vi "PSUN8731A-CTRLv3.vi"() -> ()   [LabVIEW 2017]
uses:
  Keysight N8731A conversion/Keysight N8900 Series.lvlib
  Controller subVIs/CurrentPSUSettings.vi
  <vilib>/Analysis/NI_AALPro.lvlib
  <vilib>/Analysis/6fits.llb/Curve Fitting Criteria.ctl
panel:
  in  "Quench Protection":bool
  out "Status message":string
  out "TimeData":dbl[](array[numeric])
  out "VoltData":dbl[](array[numeric])
  out "CurrData":dbl[](array[numeric])
  out "StartTime":dbl
  out "I(t)":cluster{dbl[], dbl[]}(graph)
  out "V(t)":cluster{dbl[], dbl[]}(graph)
  in  "Sweep Controller":enum32{"Sweep Mode", "Free Control Mode"}(tab)=enum."Free Control Mode"
  in  "Maximum Voltage [V]":dbl min=0.0 max=8.0 step=0.001
  in  "Maximum Current [A]":dbl min=0.0 max=400.0 step=0.1
  in  "Coil Voltage Limit [V]":dbl=0.005 min=0.0 step=0.001
  in  "Initial Voltage [V]":dbl min=0.0 max=8.0 step=0.001
  in  "Initial meas delay [ms]":u32=500 step=10
  in  "Tr meas time [s]":dbl=60.0 min=0.0
  out "Voltage offset [V]":dbl
  out "Tr [s]":dbl
  in  "Time between data points (ms)":i32=500 min=0
  out "Immediate Voltage (V)":dbl
  out "Immediate Current (A)":dbl
  in  "Voltage Set [V]":dbl min=0.0 max=8.0 step=0.001
  in  "Current Set [A]":dbl min=0.0 max=400.0 step=0.1
  in  "Voltmeter channel (6)":i32=6
  in  "End Program":bool
  in  "Stop Sweep":bool
  out "Voltmeter error message":errorcluster
  in  "Voltmeter Range (V)":dbl caption="0 for Auto range"
  in  "Voltmeter Address (16)":i16=16
  out "PSU error message":errorcluster
  in  "Start Sweep":bool
  in  "Sweepback":bool=TRUE
  in  "Power Output":bool
  in  "OC protection":bool
  in  "OV Value (10V)":dbl=10.0 min=0.5 max=10.0
  out "I(V) Graph":cluster{dbl[], dbl[]}(graph)
  in  "VISA resource name":refnum<visa-resource-name>="N8731APSU"
  in  "Filename":string caption="Leave empty to discard data.\nDon't touch during measurement"
  in  "PSU\nVoltage":bool=TRUE caption="Keithley\nVoltage"
  in  "OV protection":bool=TRUE
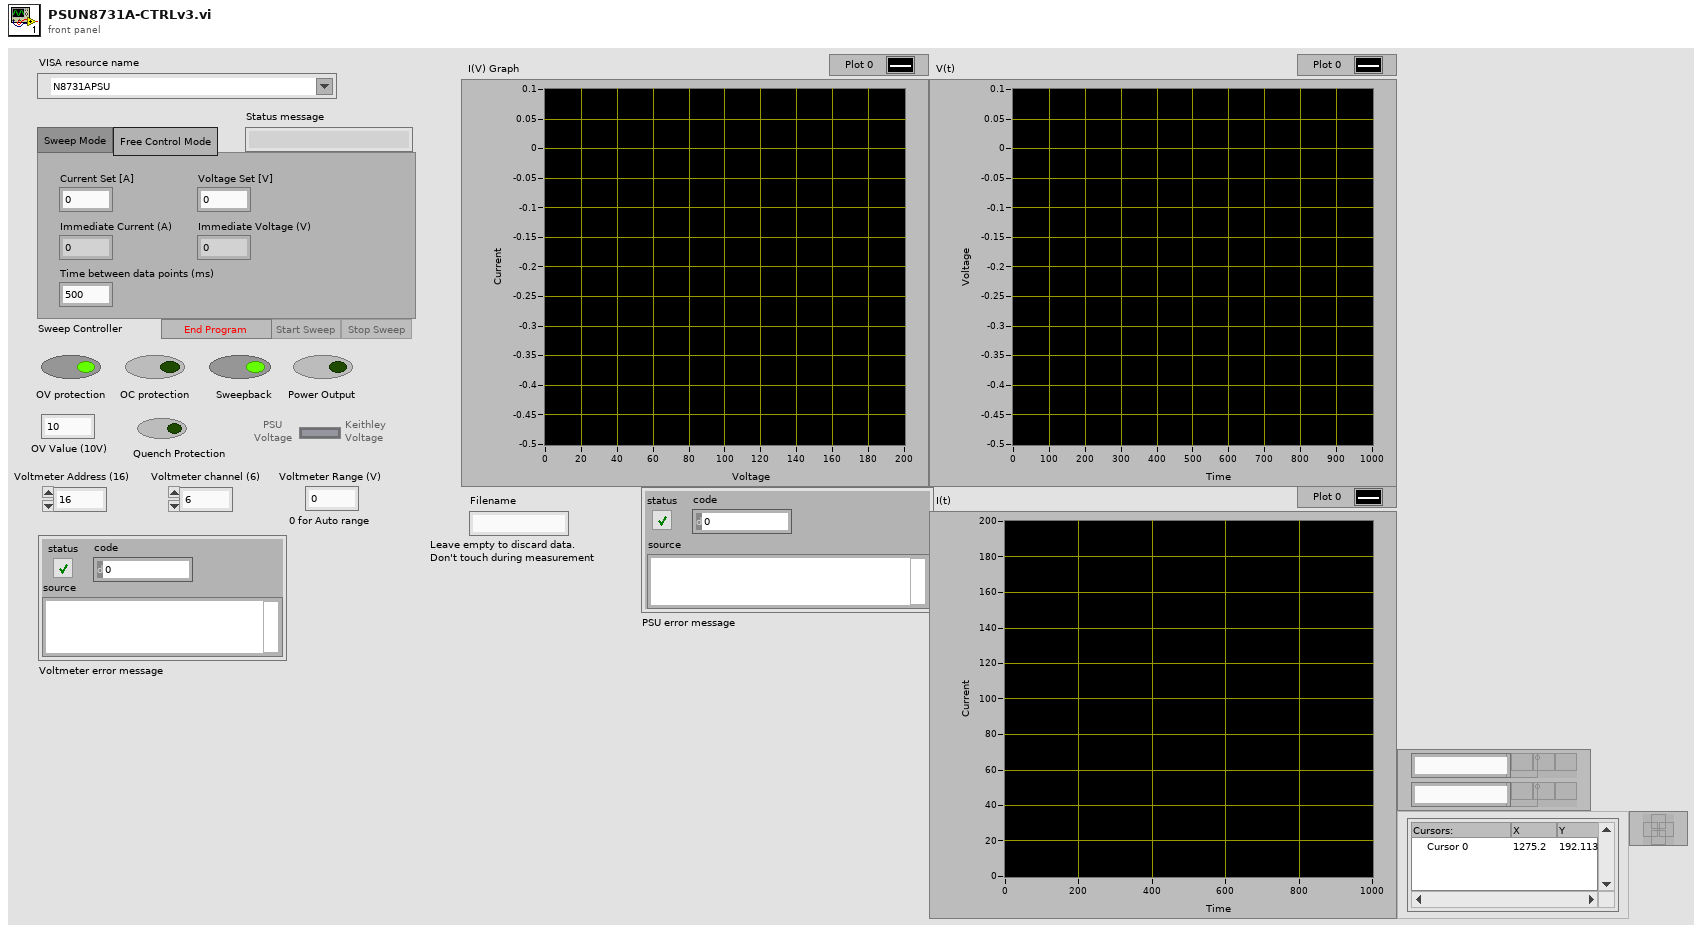
[diagram p1: front panel]
types:
  T1 = enum8{"Enabled", "Disabled", "Disabled and Grayed Out"}
  T2 = cluster{"Sweep Controller":enum32{"Sweep Mode", "Free Control Mode"}, "   PSU\nVoltage":bool}
  T3 = typedef "NI_AALPro.lvlib/Curve Fitting Criteria.ctl" = u16
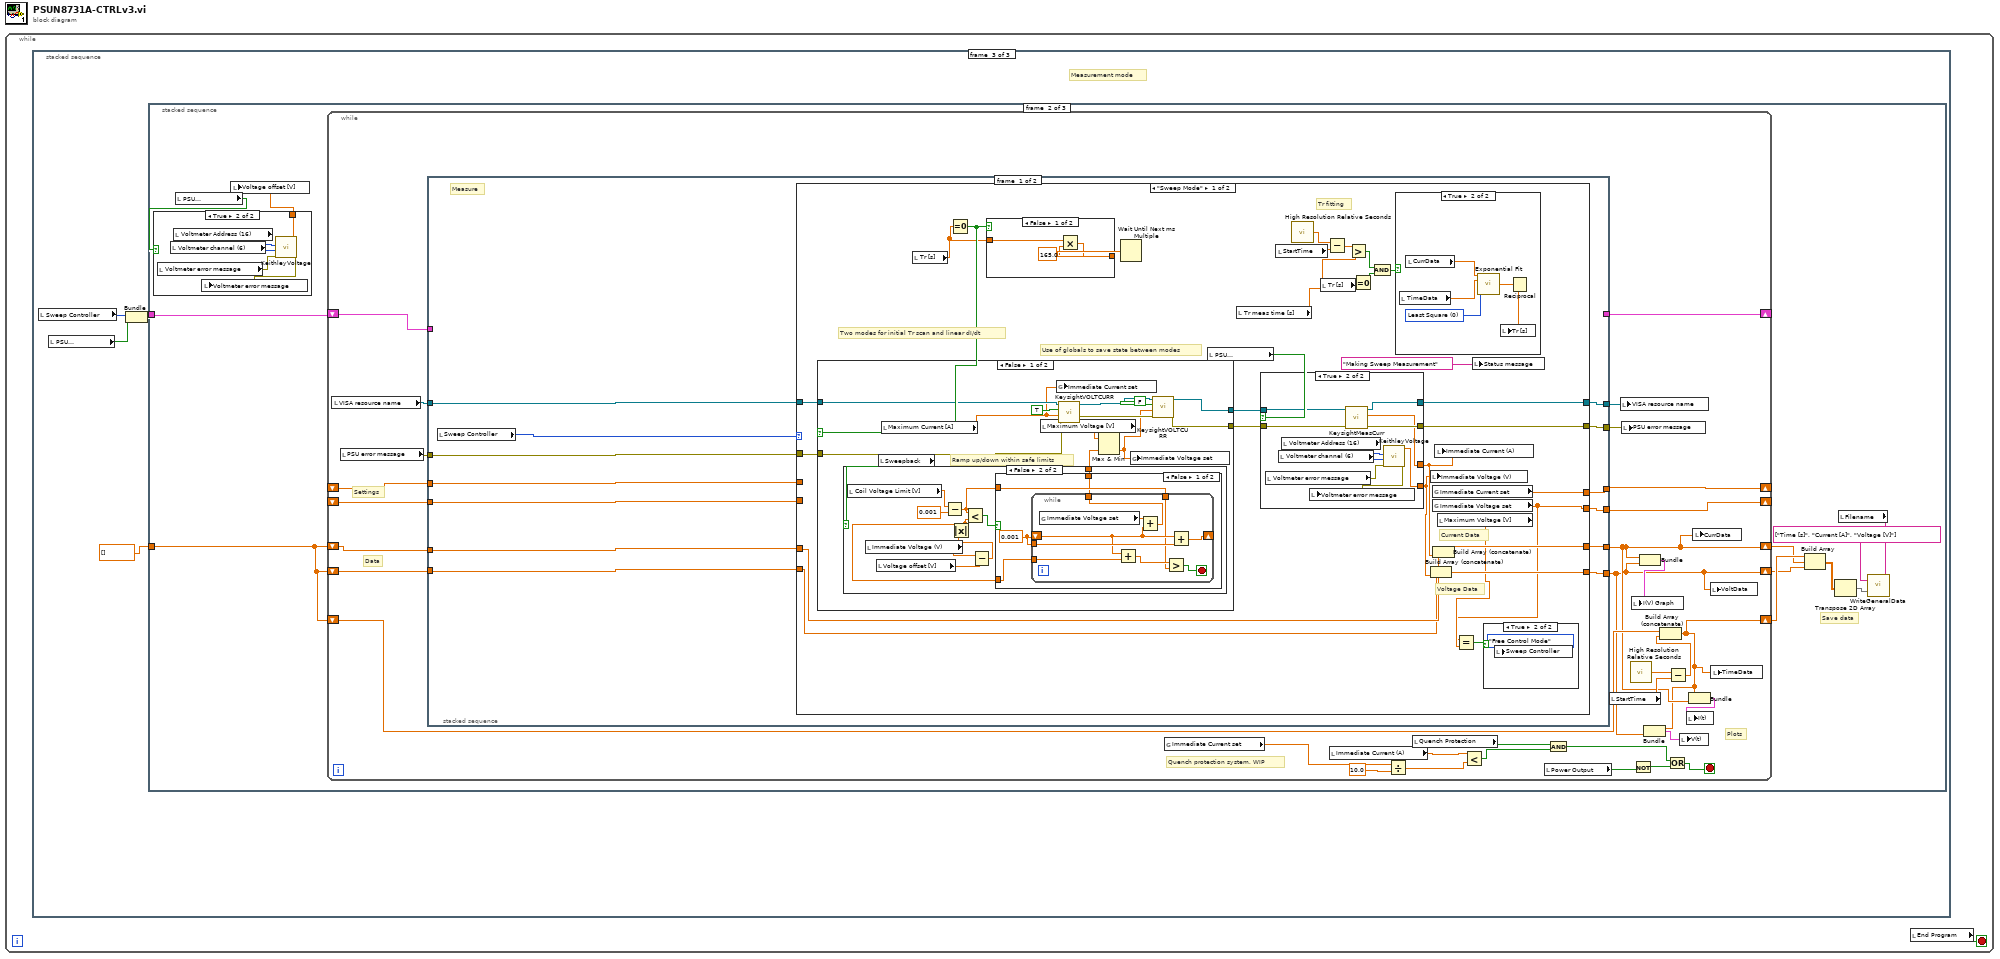
[diagram p0: block diagram]
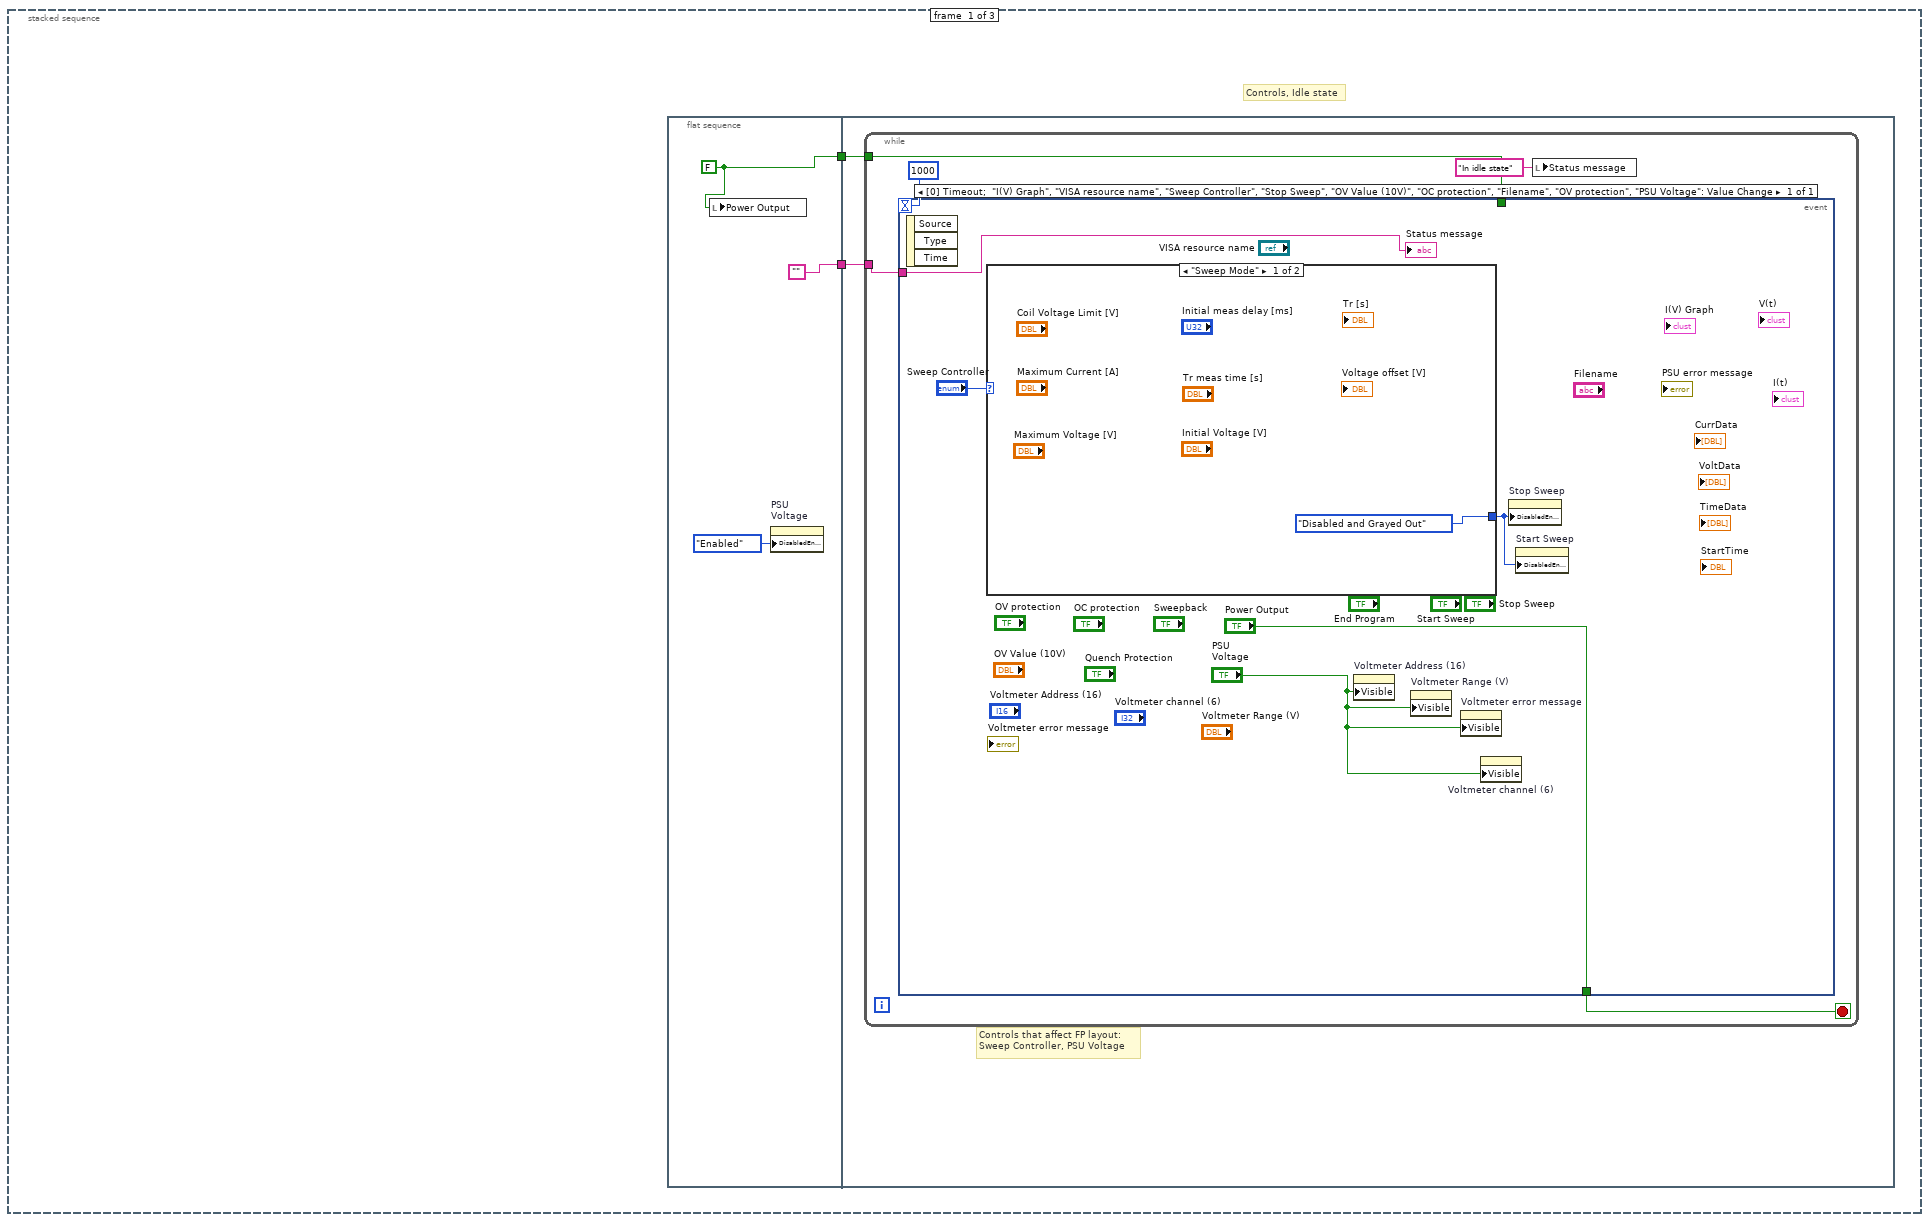
[diagram p2: hidden frame]
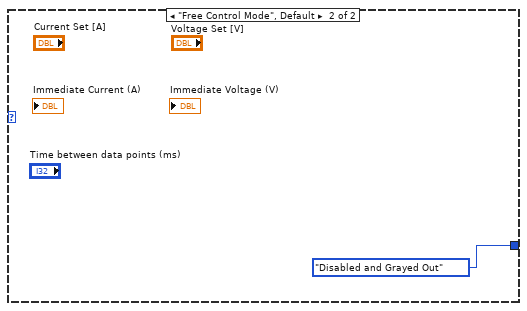
[diagram p3: hidden frame]
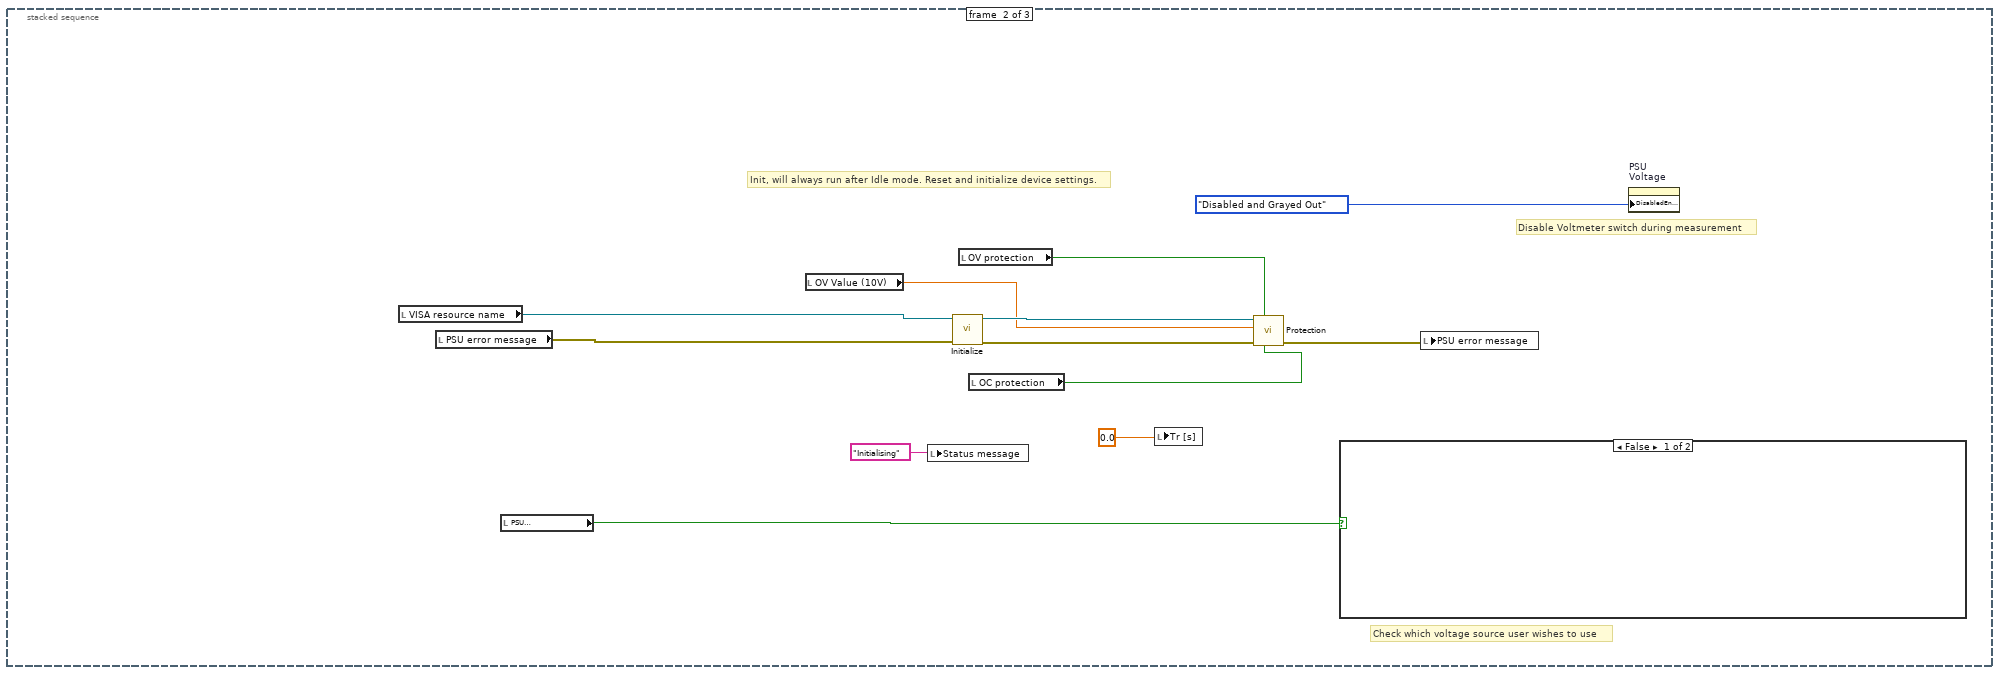
[diagram p4: hidden frame]
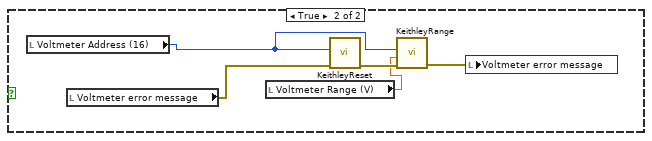
[diagram p5: hidden frame]
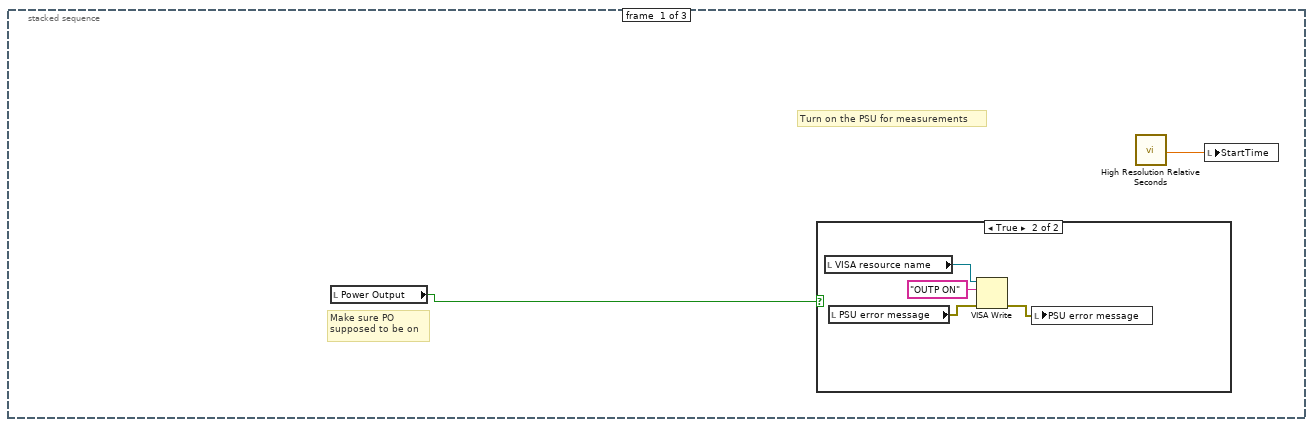
[diagram p6: hidden frame]
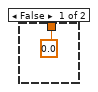
[diagram p8: hidden frame]
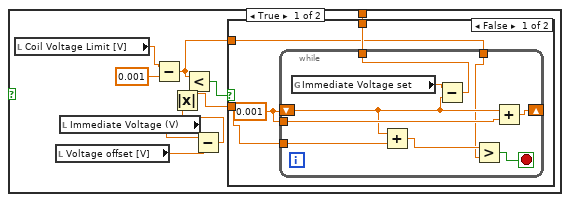
[diagram p10: hidden frame]
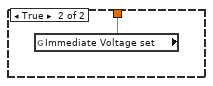
[diagram p11: hidden frame]
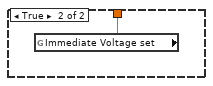
[diagram p12: hidden frame]
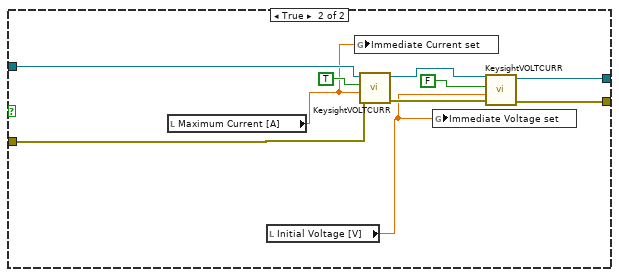
[diagram p13: hidden frame]
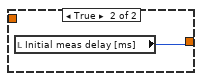
[diagram p15: hidden frame]
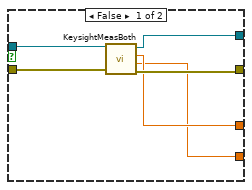
[diagram p16: hidden frame]
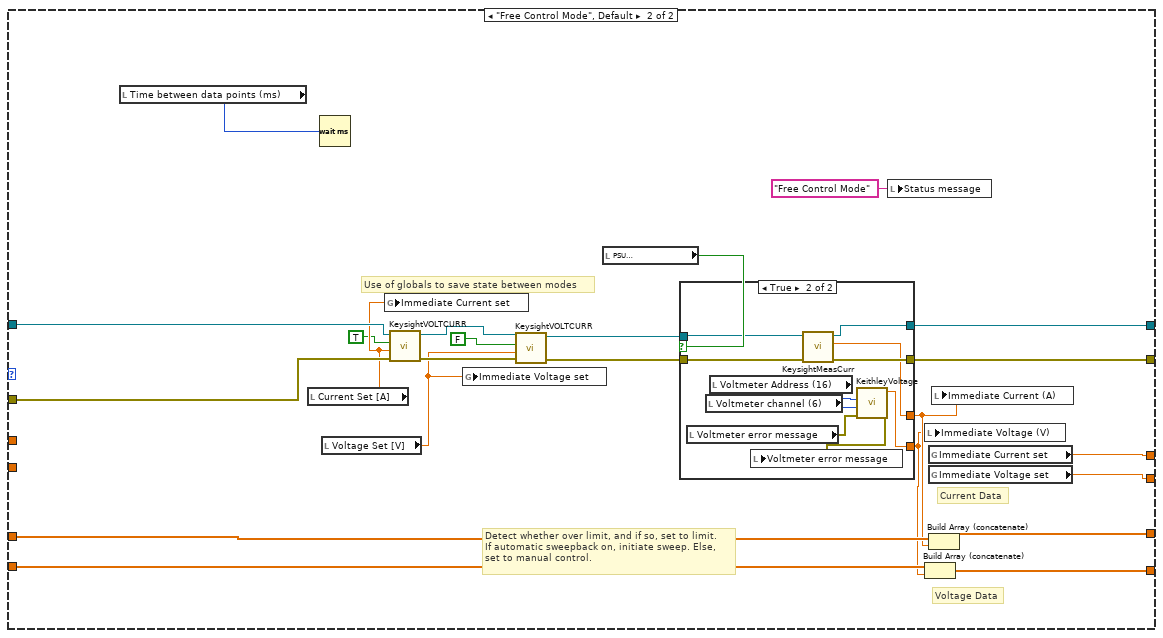
[diagram p17: hidden frame]
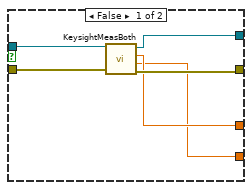
[diagram p18: hidden frame]
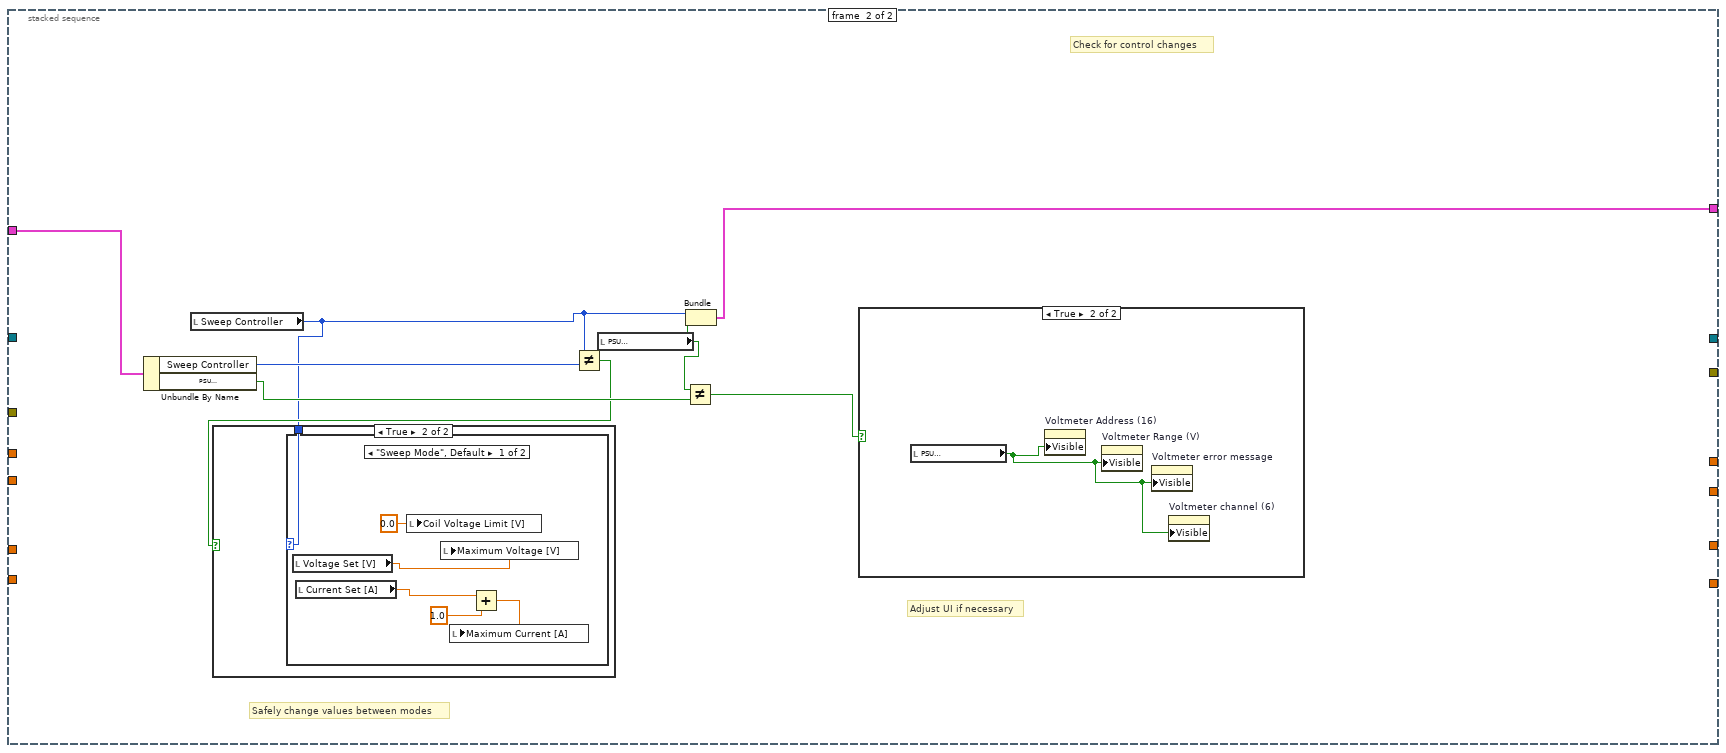
[diagram p19: hidden frame]
diagram:
  n1 = while {
    stop <- w1 stop-if-true
    n2 = stacked-sequence {
      frame #0 {
        # "Controls, Idle state"
        n3 = flat-sequence {
          tunnel: [w4] -> w3
          tunnel: ["" ("Status message")] -> w2
          tunnel: w3 -> [w8]
          tunnel: w2 -> [w7]
          frame #0 {
            w4 = FALSE ("Sweeping Back")
            n4 = local write "Power Output"(w4) -> ()
            n5 = property on="PSU\nVoltage" class="Bool (strict)"("DisabledEnum"=T1."Enabled" ("Disabled")) -> ()  [unwired: 2 in, 2 out]
          }
          frame #1 {
            # "Controls that affect FP layout:\nSweep Controller, PSU Voltage"
            n6 = while {
              tunnel: w8 -> [w11]
              tunnel: w7 -> [w10]
              stop <- w13 stop-if-true
              n7 = event shown="[0] Timeout;  \"I(V) Graph\", \"VISA resource name\", \"Sweep Controller\", \"Stop Sweep\", \"OV Value (10V)\", \"OC protection\", \"Filename\", \"OV protection\", \"PSU Voltage\": Value Change" {
                selector: _ -> [_]
                dyn-events: _ -> [_]
                timeout: 1000 -> [_]
                tunnel: ["Power Output"] -> w13
                tunnel: w11 -> [w16]
                tunnel: w10 -> [w14]
                event Timeout; "I(V) Graph", "VISA resource name", "Sweep Controller", "Stop Sweep", "OV Value (10V)", "OC protection", "Filename", "OV protection", "PSU\nVoltage": Value Change {
                  n8 = event-data() -> ()  [unwired: 1 in, 3 out]
                  n9 = case shown="\"Sweep Mode\"" "Sweep Controller" {
                    tunnel: [T1."Disabled and Grayed Out" ("Disabled") T1."Disabled and Grayed Out" ("Disabled")] -> w17
                    frame "Sweep Mode" {
                    }
                    frame "Free Control Mode", Default {
                    }
                  }
                  n10 = property on="Voltmeter Address (16)" class="DigNum (strict)"("Visible"="PSU\nVoltage") -> ()  [unwired: 2 in, 2 out]
                  n11 = property on="Voltmeter Range (V)" class="DigNum (strict)"("Visible"="PSU\nVoltage") -> ()  [unwired: 2 in, 2 out]
                  n12 = property on="Voltmeter error message" class="Clust (strict)"("Visible"="PSU\nVoltage") -> ()  [unwired: 2 in, 2 out]
                  n13 = property on="Voltmeter channel (6)" class="DigNum (strict)"("Visible"="PSU\nVoltage") -> ()  [unwired: 2 in, 2 out]
                  n14 = property on="Stop Sweep" class="Bool"("DisabledEnum"=w17) -> ()  [unwired: 2 in, 2 out]
                  n15 = property on="Start Sweep" class="Bool"("DisabledEnum"=w17) -> ()  [unwired: 2 in, 2 out]
                  "Status message" <- w14
                }
              }
              n16 = local write "Status message"("In idle state" ("Status message")) -> ()
            }
          }
        }
      }
      frame #1 {
        # "Check which voltage source user wishes to use"
        # "Disable Voltmeter switch during measurement"
        # "Init, will always run after Idle mode. Reset and initialize device settings."
        n17 = local read "VISA resource name"() -> (w31:refnum<visa-resource-name>)
        n18 = local read "PSU error message"() -> (w26:errorcluster)
        n19 = local read "PSU\nVoltage"() -> (w25:bool)
        n20 = local read "OV Value (10V)"() -> (w30:dbl)
        n21 = local write "Status message"("Initialising" ("Status message")) -> ()
        n22 = call "Initialize.vi"("error in (no error)"=w26, "VISA resource name"=w31) -> ("error out"=w32:errorcluster, "VISA resource name out"=w33:refnum<visa-resource-name>)  [unwired: 8 in]
        n23 = local read "OV protection"() -> (w28:bool)
        n24 = local read "OC protection"() -> (w29:bool)
        n25 = local write "Tr [s]"(0.0 ("Tr")) -> ()
        n26 = call "Protection.vi"("OC protection"=w29, "OV protection"=w28, "error in (no error)"=w32, "OV Value (10V)"=w30, "VISA resource name"=w33) -> ("error out"=w27:errorcluster)  [unwired: 5 in, 1 out]
        n27 = case shown="False" w25 {
          frame False {
          }
          frame True {
            n28 = local read "Voltmeter Address (16)"() -> (w34:i16)
            n29 = local read "Voltmeter error message"() -> (w36:errorcluster)
            n30 = local read "Voltmeter Range (V)"() -> (w35:dbl)
            n31 = call "KeithleyReset.vi"("error in"=w36, "address (16)"=w34) -> ("error out"=w37:errorcluster)  [unwired: 9 in]
            n32 = call "KeithleyRange.vi"("error in"=w37, "Range (V)/Auto(0)"=w35, "address (16)"=w34) -> ("error out"=w38:errorcluster)  [unwired: 8 in]
            n33 = local write "Voltmeter error message"(w38) -> ()
          }
        }
        n34 = local write "PSU error message"(w27) -> ()
        n35 = property on="PSU\nVoltage" class="Bool (strict)"("DisabledEnum"=T1."Disabled and Grayed Out" ("Disabled")) -> ()  [unwired: 2 in, 2 out]
      }
      frame #2 {
        # "Measurement mode"
        n36 = local read "Sweep Controller"() -> (w42:enum32{"Sweep Mode", "Free Control Mode"})
        n37 = local read "PSU\nVoltage"() -> (w41:bool)
        n38 = Bundle("Sweep Controller"=w42, "PSU\nVoltage"=w41) -> (w40:T2)  [unwired: 1 in]
        n39 = stacked-sequence {
          tunnel: w40 -> [_ w59 _]
          tunnel: dbl[] [] -> [_ w58 _]
          frame #0 {
            # "Make sure PO\nsupposed to be on"
            # "Turn on the PSU for measurements"
            n40 = local read "Power Output"() -> (w44:bool)
            n41 = case shown="True" w44 {
              frame False {
              }
              frame True {
                n42 = local read "VISA resource name"() -> (w47:refnum<visa-resource-name>)
                n43 = local read "PSU error message"() -> (w46:errorcluster)
                n44 = VISA Write(VISA resource name=w47, write buffer="OUTP ON", error in (no error)=w46) -> (error out=w45:errorcluster)  [unwired: 2 out]
                n45 = local write "PSU error message"(w45) -> ()
              }
            }
            n46 = call <vilib>:"High Resolution Relative Seconds.vi"() -> ("relative seconds"=w43:dbl)
            n47 = local write "StartTime"(w43) -> ()
          }
          frame #1 {
            # "Save data"
            n48 = local read "PSU\nVoltage"() -> (w57:bool)
            n49 = case shown="True" w57 {
              tunnel: [0.0 ("Voltage") w61] -> w56
              frame False {
              }
              frame True {
                n50 = local read "Voltmeter error message"() -> (w63:errorcluster)
                n51 = local read "Voltmeter channel (6)"() -> (w65:i32)
                n52 = local read "Voltmeter Address (16)"() -> (w64:i16)
                n53 = call "KeithleyVoltage.vi"("error in"=w63, "channel (6)"=w65, "address (16)"=w64) -> ("error out"=w62:errorcluster, "Voltage"=w61:dbl)  [unwired: 7 in]
                n54 = local write "Voltmeter error message"(w62) -> ()
              }
            }
            n55 = local write "Voltage offset [V]"(w56) -> ()
            n56 = while {
              shift-right: [w67] -> _
              shift-left: w59 -> [w97]
              shift-right: [w88] -> _
              shift-left: _ -> [w86]
              shift-right: [w89] -> _
              shift-left: _ -> [w94]
              shift-right: [w70] -> w52
              shift-left: w58 -> [w91]
              shift-right: [w69] -> w51
              shift-left: w58 -> [w90]
              shift-right: [w68] -> w53
              shift-left: w58 -> [w84]
              stop <- w71 stop-if-true
              # "Plots"
              # "Quench protection system, WIP"
              # "Data"
              # "Settings"
              n57 = local read "VISA resource name"() -> (w96:refnum<visa-resource-name>)
              n58 = local read "PSU error message"() -> (w95:errorcluster)
              n59 = stacked-sequence {
                tunnel: w97 -> [_ w280]
                tunnel: w96 -> [w109 _]
                tunnel: w95 -> [w108 _]
                tunnel: w94 -> [w107 _]
                tunnel: [w106 _] -> w93
                tunnel: [w105 _] -> w92
                tunnel: w91 -> [w104 _]
                tunnel: [w103 _] -> w70
                tunnel: w90 -> [w102 _]
                tunnel: [w101 _] -> w69
                tunnel: [w100 _] -> w89
                tunnel: [w99 _] -> w88
                tunnel: w86 -> [w98 _]
                tunnel: [_ w276] -> w67
                frame #0 {
                  # "Measure"
                  n60 = local read "Sweep Controller"() -> (w110:enum32{"Sweep Mode", "Free Control Mode"})
                  n61 = case shown="\"Sweep Mode\"" w110 {
                    tunnel: w109 -> [w139 w257]
                    tunnel: w108 -> [w138 w256]
                    tunnel: w107 -> [_ _]
                    tunnel: [w137 w255] -> w106
                    tunnel: [w136 w254] -> w105
                    tunnel: w104 -> [w135 w253]
                    tunnel: [w134 w252] -> w103
                    tunnel: w102 -> [w117 w251]
                    tunnel: [w133 w250] -> w101
                    tunnel: [w127 w238] -> w100
                    tunnel: [w111 w237] -> w99
                    tunnel: w98 -> [_ _]
                    frame "Sweep Mode" {
                      # "Tr fitting"
                      # "Two modes for initial Tr scan and linear dI/dt"
                      # "Use of globals to save state between modes"
                      # "Voltage Data"
                      # "Current Data"
                      n62 = local read "Tr [s]"() -> (w116:dbl)
                      n63 = Equal To 0?(x=w116) -> (x = 0?=w118:bool)
                      n64 = case shown="False" w118 {
                        tunnel: w139 -> [w153 w209]
                        tunnel: w138 -> [w152 w208]
                        tunnel: [w147 w203] -> w131
                        tunnel: [w146 w202] -> w130
                        frame False {
                          # "Ramp up/down within safe limits"
                          n65 = local read "Sweepback"() -> (w144:bool)
                          n66 = case shown="False" w144 {
                            tunnel: [w162 w185] -> w142
                            frame True {
                              n67 = local read "Coil Voltage Limit [V]"() -> (w157:dbl)
                              n68 = local read "Voltage offset [V]"() -> (w160:dbl)
                              n69 = local read "Immediate Voltage (V)"() -> (w161:dbl)
                              n70 = Subtract(x=w157, y=0.001) -> (x-y=w155:dbl)
                              n71 = Subtract(x=w161, y=w160) -> (x-y=w156:dbl)
                              n72 = Absolute Value(x=w156) -> (abs(x)=w154:dbl)
                              n73 = Less?(x=w155, y=w154) -> (x < y?=w159:bool)
                              n74 = case shown="False" w159 {
                                tunnel: [w165 w176] -> w162
                                tunnel: w155 -> [w164 _]
                                tunnel: w154 -> [w163 _]
                                frame False {
                                w166 = 0.001 ("y")
                                n75 = while {
                                shift-right: [w174] -> _
                                shift-left: w166 -> [w169]
                                tunnel: w166 -> [w173]
                                tunnel: [w172] -> w165
                                tunnel: w164 -> [w167]
                                tunnel: w163 -> [w170]
                                stop <- w175 stop-if-true
                                n76 = global read "CurrentPSUSettings.vi" "Immediate Voltage set"() -> (w171:dbl)
                                n77 = Add(x=w169, y=w170) -> (x+y=w168:dbl)
                                n78 = Subtract(x=w171, y=w169) -> (x-y=w172:dbl)
                                n79 = Greater?(x=w168, y=w167) -> (0:w175:bool)
                                n80 = Add(x=w169, y=w173) -> (x+y=w174:dbl)
                                }
                                }
                                frame True {
                                n81 = global read "CurrentPSUSettings.vi" "Immediate Voltage set"() -> (w176:dbl)
                                }
                              }
                            }
                            frame False {
                              n82 = local read "Coil Voltage Limit [V]"() -> (w180:dbl)
                              n83 = local read "Immediate Voltage (V)"() -> (w184:dbl)
                              n84 = local read "Voltage offset [V]"() -> (w183:dbl)
                              n85 = Subtract(x=w180, y=0.001) -> (x-y=w178:dbl)
                              n86 = Subtract(x=w184, y=w183) -> (x-y=w179:dbl)
                              n87 = Absolute Value(x=w179) -> (abs(x)=w177:dbl)
                              n88 = Less?(x=w178, y=w177) -> (x < y?=w182:bool)
                              n89 = case shown="False" w182 {
                                tunnel: [w187 w199] -> w185
                                tunnel: w178 -> [w189 _]
                                tunnel: w177 -> [w186 _]
                                frame False {
                                w188 = 0.001 ("y")
                                n90 = while {
                                shift-right: [w197] -> _
                                shift-left: w188 -> [w193]
                                tunnel: w189 -> [w190]
                                tunnel: w188 -> [w196]
                                tunnel: [w195] -> w187
                                tunnel: w186 -> [w192]
                                stop <- w198 stop-if-true
                                n91 = global read "CurrentPSUSettings.vi" "Immediate Voltage set"() -> (w194:dbl)
                                n92 = Add(x=w193, y=w192) -> (x+y=w191:dbl)
                                n93 = Add(x=w194, y=w193) -> (x+y=w195:dbl)
                                n94 = Greater?(x=w191, y=w190) -> (0:w198:bool)
                                n95 = Add(x=w193, y=w196) -> (x+y=w197:dbl)
                                }
                                }
                                frame True {
                                n96 = global read "CurrentPSUSettings.vi" "Immediate Voltage set"() -> (w199:dbl)
                                }
                              }
                            }
                          }
                          n97 = local read "Maximum Current [A]"() -> (w145:dbl)
                          n98 = local read "Maximum Voltage [V]"() -> (w143:dbl)
                          n99 = global write "CurrentPSUSettings.vi" "Immediate Current set"(w145) -> ()
                          n100 = call "KeysightVOLTCURR.vi"("error in (no error)"=w152, "CURR/VOLT (A/V)"=w145, "CURR (1)/VOLT (0)"=TRUE, "VISA resource name"=w153) -> ("error out"=w148:errorcluster, "VISA resource name out"=w149:refnum<visa-resource-name>)  [unwired: 6 in]
                          n101 = Max & Min(x=w143, y=w142) -> (min(x,y)=w141:dbl)  [unwired: 1 out]
                          n102 = global write "CurrentPSUSettings.vi" "Immediate Voltage set"(w141) -> ()
                          n103 = call "KeysightVOLTCURR.vi"("error in (no error)"=w148, "CURR/VOLT (A/V)"=w141, "CURR (1)/VOLT (0)"=FALSE, "VISA resource name"=w149) -> ("error out"=w146:errorcluster, "VISA resource name out"=w147:refnum<visa-resource-name>)  [unwired: 6 in]
                        }
                        frame True {
                          n104 = local read "Maximum Current [A]"() -> (w201:dbl)
                          n105 = local read "Initial Voltage [V]"() -> (w200:dbl)
                          n106 = global write "CurrentPSUSettings.vi" "Immediate Current set"(w201) -> ()
                          n107 = call "KeysightVOLTCURR.vi"("error in (no error)"=w208, "CURR/VOLT (A/V)"=w201, "CURR (1)/VOLT (0)"=TRUE, "VISA resource name"=w209) -> ("error out"=w204:errorcluster, "VISA resource name out"=w205:refnum<visa-resource-name>)  [unwired: 6 in]
                          n108 = global write "CurrentPSUSettings.vi" "Immediate Voltage set"(w200) -> ()
                          n109 = call "KeysightVOLTCURR.vi"("error in (no error)"=w204, "CURR/VOLT (A/V)"=w200, "CURR (1)/VOLT (0)"=FALSE, "VISA resource name"=w205) -> ("error out"=w202:errorcluster, "VISA resource name out"=w203:refnum<visa-resource-name>)  [unwired: 6 in]
                        }
                      }
                      n110 = case shown="False" w118 {
                        tunnel: [w216 w218] -> w126
                        tunnel: w116 -> [w215 _]
                        frame False {
                          n111 = Multiply(x=w215, y=165.0 ("Tr")) -> (x*y=w216:dbl)
                        }
                        frame True {
                          n112 = local read "Initial meas delay [ms]"() -> (w218:u32)
                        }
                      }
                      n113 = Wait Until Next ms Multiple(millisecond multiple=w126) -> ()  [unwired: 1 out]
                      n114 = local read "PSU\nVoltage"() -> (w132:bool)
                      n115 = local read "Tr meas time [s]"() -> (w115:dbl)
                      n116 = case shown="True" w132 {
                        tunnel: w131 -> [w224 w234]
                        tunnel: w130 -> [w223 w233]
                        tunnel: [w222 w228] -> w137
                        tunnel: [w221 w227] -> w136
                        tunnel: [w220 w226] -> w129
                        tunnel: [w219 w225] -> w128
                        frame False {
                          n117 = call "KeysightMeasBoth.vi"("error in (no error)"=w223, "VISA resource name"=w224) -> ("error out"=w221:errorcluster, "VOLT"=w219:dbl, "CURR"=w220:dbl, "VISA resource name out"=w222:refnum<visa-resource-name>)  [unwired: 6 in]
                        }
                        frame True {
                          n118 = local read "Voltmeter error message"() -> (w230:errorcluster)
                          n119 = local read "Voltmeter channel (6)"() -> (w232:i32)
                          n120 = local read "Voltmeter Address (16)"() -> (w231:i16)
                          n121 = call "KeysightMeasCurr.vi"("error in (no error)"=w233, "VISA resource name"=w234) -> ("error out"=w227:errorcluster, "CURR"=w226:dbl, "VISA resource name out"=w228:refnum<visa-resource-name>)  [unwired: 7 in]
                          n122 = call "KeithleyVoltage.vi"("error in"=w230, "channel (6)"=w232, "address (16)"=w231) -> ("error out"=w229:errorcluster, "Voltage"=w225:dbl)  [unwired: 7 in]
                          n123 = local write "Voltmeter error message"(w229) -> ()
                        }
                      }
                      n124 = local read "StartTime"() -> (w124:dbl)
                      n125 = call <vilib>:"High Resolution Relative Seconds.vi"() -> ("relative seconds"=w125:dbl)
                      n126 = local read "Tr [s]"() -> (w121:dbl)
                      n127 = Subtract(x=w125, y=w124) -> (x-y=w123:dbl)
                      n128 = Greater?(x=w123, y=w115) -> (0:w119:bool)
                      n129 = Equal To 0?(x=w121) -> (x = 0?=w120:bool)
                      n130 = And(x=w119, y=w120) -> (x .and. y?=w122:bool)
                      n131 = case shown="True" w122 {
                        frame False {
                        }
                        frame True {
                          w212 = T3 0 items=["Least Square", "Least Absolute Residual", "Bisquare"] ("method")
                          n132 = local read "TimeData"() -> (w213:dbl[])
                          n133 = local read "CurrData"() -> (w214:dbl[])
                          n134 = call <vilib>:"Exponential Fit.vi"("Y"=w214, "X"=w213, "method"=w212) -> ("damping"=w210:dbl)  [unwired: 7 in, 5 out]
                          n135 = Reciprocal(x=w210) -> (1/x=w211:dbl)
                          n136 = local write "Tr [s]"(w211) -> ()
                        }
                      }
                      n137 = local write "Immediate Voltage (V)"(w128) -> ()
                      n138 = Build Array (concatenate)(w117, w128) -> (w133:dbl[])
                      n139 = global read "CurrentPSUSettings.vi" "Immediate Current set"() -> (w127:dbl)
                      n140 = global read "CurrentPSUSettings.vi" "Immediate Voltage set"() -> (w111:dbl)
                      n141 = Build Array (concatenate)(w135, w129) -> (w134:dbl[])
                      n142 = local write "Immediate Current (A)"(w129) -> ()
                      n143 = local read "Maximum Voltage [V]"() -> (w112:dbl)
                      n144 = Equal?(x=w111, y=w112) -> (x = y?=w113:bool)
                      n145 = local write "Status message"("Making Sweep Measurement" ("Status message")) -> ()
                      n146 = case shown="True" w113 {
                        frame False {
                        }
                        frame True {
                          n147 = local write "Sweep Controller"(enum32{"Sweep Mode", "Free Control Mode"}."Free Control Mode" ("Sweep Controller")) -> ()
                        }
                      }
                    }
                    frame "Free Control Mode", Default {
                      # "Use of globals to save state between modes"
                      # "Detect whether over limit, and if so, set to limit.\nIf automatic sweepback on, initiate sweep. Else,\nset to manual control."
                      # "Voltage Data"
                      # "Current Data"
                      n148 = local read "Time between data points (ms)"() -> (w236:i32)
                      n149 = local read "Current Set [A]"() -> (w249:dbl)
                      n150 = Wait (ms)(milliseconds to wait=w236) -> ()  [unwired: 1 out]
                      n151 = local read "Voltage Set [V]"() -> (w240:dbl)
                      n152 = global write "CurrentPSUSettings.vi" "Immediate Current set"(w249) -> ()
                      n153 = call "KeysightVOLTCURR.vi"("error in (no error)"=w256, "CURR/VOLT (A/V)"=w249, "CURR (1)/VOLT (0)"=TRUE, "VISA resource name"=w257) -> ("error out"=w245:errorcluster, "VISA resource name out"=w246:refnum<visa-resource-name>)  [unwired: 6 in]
                      n154 = global write "CurrentPSUSettings.vi" "Immediate Voltage set"(w240) -> ()
                      n155 = call "KeysightVOLTCURR.vi"("error in (no error)"=w245, "CURR/VOLT (A/V)"=w240, "CURR (1)/VOLT (0)"=FALSE, "VISA resource name"=w246) -> ("error out"=w242:errorcluster, "VISA resource name out"=w243:refnum<visa-resource-name>)  [unwired: 6 in]
                      n156 = local read "PSU\nVoltage"() -> (w244:bool)
                      n157 = case shown="True" w244 {
                        tunnel: w243 -> [w263 w273]
                        tunnel: w242 -> [w262 w272]
                        tunnel: [w261 w267] -> w255
                        tunnel: [w260 w266] -> w254
                        tunnel: [w259 w265] -> w241
                        tunnel: [w258 w264] -> w239
                        frame False {
                          n158 = call "KeysightMeasBoth.vi"("error in (no error)"=w262, "VISA resource name"=w263) -> ("error out"=w260:errorcluster, "VOLT"=w258:dbl, "CURR"=w259:dbl, "VISA resource name out"=w261:refnum<visa-resource-name>)  [unwired: 6 in]
                        }
                        frame True {
                          n159 = local read "Voltmeter error message"() -> (w269:errorcluster)
                          n160 = local read "Voltmeter channel (6)"() -> (w271:i32)
                          n161 = local read "Voltmeter Address (16)"() -> (w270:i16)
                          n162 = call "KeysightMeasCurr.vi"("error in (no error)"=w272, "VISA resource name"=w273) -> ("error out"=w266:errorcluster, "CURR"=w265:dbl, "VISA resource name out"=w267:refnum<visa-resource-name>)  [unwired: 7 in]
                          n163 = call "KeithleyVoltage.vi"("error in"=w269, "channel (6)"=w271, "address (16)"=w270) -> ("error out"=w268:errorcluster, "Voltage"=w264:dbl)  [unwired: 7 in]
                          n164 = local write "Voltmeter error message"(w268) -> ()
                        }
                      }
                      n165 = local write "Status message"("Free Control Mode" ("Status message")) -> ()
                      n166 = local write "Immediate Voltage (V)"(w239) -> ()
                      n167 = Build Array (concatenate)(w251, w239) -> (w250:dbl[])
                      n168 = global read "CurrentPSUSettings.vi" "Immediate Current set"() -> (w238:dbl)
                      n169 = global read "CurrentPSUSettings.vi" "Immediate Voltage set"() -> (w237:dbl)
                      n170 = Build Array (concatenate)(w253, w241) -> (w252:dbl[])
                      n171 = local write "Immediate Current (A)"(w241) -> ()
                    }
                  }
                }
                frame #1 {
                  # "Safely change values between modes"
                  # "Adjust UI if necessary"
                  # "Check for control changes"
                  n172 = Unbundle By Name(w280) -> ("Sweep Controller"=w281:enum32{"Sweep Mode", "Free Control Mode"}, "PSU\nVoltage"=w278:bool)
                  n173 = local read "Sweep Controller"() -> (w274:enum32{"Sweep Mode", "Free Control Mode"})
                  n174 = Not Equal?(x=w274, y=w281) -> (x != y?=w275:bool)
                  n175 = case shown="True" w275 {
                    tunnel: w274 -> [_ w282]
                    frame False {
                    }
                    frame True {
                      n176 = case shown="\"Sweep Mode\", Default" w282 {
                        frame "Sweep Mode", Default {
                          n177 = local read "Voltage Set [V]"() -> (w283:dbl)
                          n178 = local read "Current Set [A]"() -> (w284:dbl)
                          n179 = local write "Coil Voltage Limit [V]"(0.0 ("Coil Voltage Limit [V]")) -> ()
                          n180 = local write "Maximum Voltage [V]"(w283) -> ()
                          n181 = Add(x=w284, y=1.0) -> (x+y=w285:dbl)
                          n182 = local write "Maximum Current [A]"(w285) -> ()
                        }
                        frame "Free Control Mode" {
                          n183 = global read "CurrentPSUSettings.vi" "Immediate Current set"() -> (w290:dbl)
                          n184 = global read "CurrentPSUSettings.vi" "Immediate Voltage set"() -> (w291:dbl)
                          n185 = local read "Tr [s]"() -> (w289:dbl)
                          n186 = Not Equal To 0?(x=w289) -> (x != 0?=w288:bool)
                          n187 = case shown="True" w288 {
                            tunnel: w289 -> [_ w293]
                            frame False {
                            }
                            frame True {
                              n188 = Multiply(x=w293, y=1000.0) -> (x*y=w292:dbl)
                              n189 = local write "Time between data points (ms)"(w292) -> ()
                            }
                          }
                          n190 = local write "Current Set [A]"(w290) -> ()
                          n191 = local write "Voltage Set [V]"(w291) -> ()
                        }
                      }
                    }
                  }
                  n192 = local read "PSU\nVoltage"() -> (w279:bool)
                  n193 = Not Equal?(x=w279, y=w278) -> (x != y?=w277:bool)
                  n194 = Bundle("Sweep Controller"=w274, "PSU\nVoltage"=w279) -> (w276:T2)  [unwired: 1 in]
                  n195 = case shown="True" w277 {
                    frame False {
                    }
                    frame True {
                      n196 = local read "PSU\nVoltage"() -> (w295:bool)
                      n197 = property on="Voltmeter Address (16)" class="DigNum (strict)"("Visible"=w295) -> ()  [unwired: 2 in, 2 out]
                      n198 = property on="Voltmeter Range (V)" class="DigNum (strict)"("Visible"=w295) -> ()  [unwired: 2 in, 2 out]
                      n199 = property on="Voltmeter error message" class="Clust (strict)"("Visible"=w295) -> ()  [unwired: 2 in, 2 out]
                      n200 = property on="Voltmeter channel (6)" class="DigNum (strict)"("Visible"=w295) -> ()  [unwired: 2 in, 2 out]
                    }
                  }
                }
              }
              n201 = global read "CurrentPSUSettings.vi" "Immediate Current set"() -> (w76:dbl)
              n202 = local read "Immediate Current (A)"() -> (w77:dbl)
              n203 = Divide(x=w76, y=10.0) -> (x/y=w74:dbl)
              n204 = local read "Quench Protection"() -> (w66:bool)
              n205 = Less?(x=w77, y=w74) -> (x < y?=w78:bool)
              n206 = local read "Power Output"() -> (w85:bool)
              n207 = And(x=w66, y=w78) -> (x .and. y?=w72:bool)
              n208 = local read "StartTime"() -> (w82:dbl)
              n209 = local write "VISA resource name"(w93) -> ()
              n210 = local write "PSU error message"(w92) -> ()
              n211 = call <vilib>:"High Resolution Relative Seconds.vi"() -> ("relative seconds"=w83:dbl)
              n212 = Not(x=w85) -> (.not. x?=w73:bool)
              n213 = Bundle(w70, w69) -> (w87:cluster{dbl[], dbl[]})  [unwired: 1 in]
              n214 = local write "I(V) Graph"(w87) -> ()
              n215 = Or(x=w72, y=w73) -> (x .or. y?=w71:bool)
              n216 = Subtract(x=w83, y=w82) -> (x-y=w81:dbl)
              n217 = Build Array (concatenate)(w84, w81) -> (w68:dbl[])
              n218 = Bundle(w68, w69) -> (w80:cluster{dbl[], dbl[]})  [unwired: 1 in]
              n219 = local write "V(t)"(w80) -> ()
              n220 = Bundle(w68, w70) -> (w79:cluster{dbl[], dbl[]})  [unwired: 1 in]
              n221 = local write "I(t)"(w79) -> ()
              n222 = local write "CurrData"(w70) -> ()
              n223 = local write "VoltData"(w69) -> ()
              n224 = local write "TimeData"(w68) -> ()
            }
            n225 = Build Array(w53, w52, w51) -> (w49:dbl[][])
            n226 = Transpose 2D Array(2D array=w49) -> (transposed array=w50:dbl[][])
            n227 = local read "Filename"() -> (w55:string)
            n228 = call "WriteGeneralData.vi"("filename (discard if empty)"=w55, "Array"=w50, "Column name array"=string[] ["Time [s]", "Current [A]", "Voltage [V]"]) -> ()
          }
          frame #2 {
            # "Turn off PSU after measurements"
            n229 = local read "VISA resource name"() -> (w301:refnum<visa-resource-name>)
            n230 = local read "PSU error message"() -> (w300:errorcluster)
            n231 = VISA Write(VISA resource name=w301, write buffer="OUTP OFF", error in (no error)=w300) -> (VISA resource name out=w298:refnum<visa-resource-name>, error out=w297:errorcluster)  [unwired: 1 out]
            n232 = call "Close.vi"("error in (no error)"=w297, "VISA resource name"=w298) -> ("error out"=w296:errorcluster)  [unwired: 9 in]
            n233 = local write "PSU error message"(w296) -> ()
          }
        }
      }
    }
    n234 = local read "End Program"() -> (w1:bool)
  }
